vi "Main.vi"() -> ()   [LabVIEW 2017]
panel:
  out "max V":dbl
  out "Loop Iterations":i32
  out "Displacement Array":dbl[](array[numeric])
  out "Velocity Array":dbl[](array[numeric])
  out "Accel Array":dbl[](array[numeric])
  out "Displacement":dbl[](graph)
  out "Velocity":dbl[](graph)
  out "Acceleration":dbl[](graph)
  out "Motion Planning Outputs":T1
  in  "Motion Planning Inputs":T2
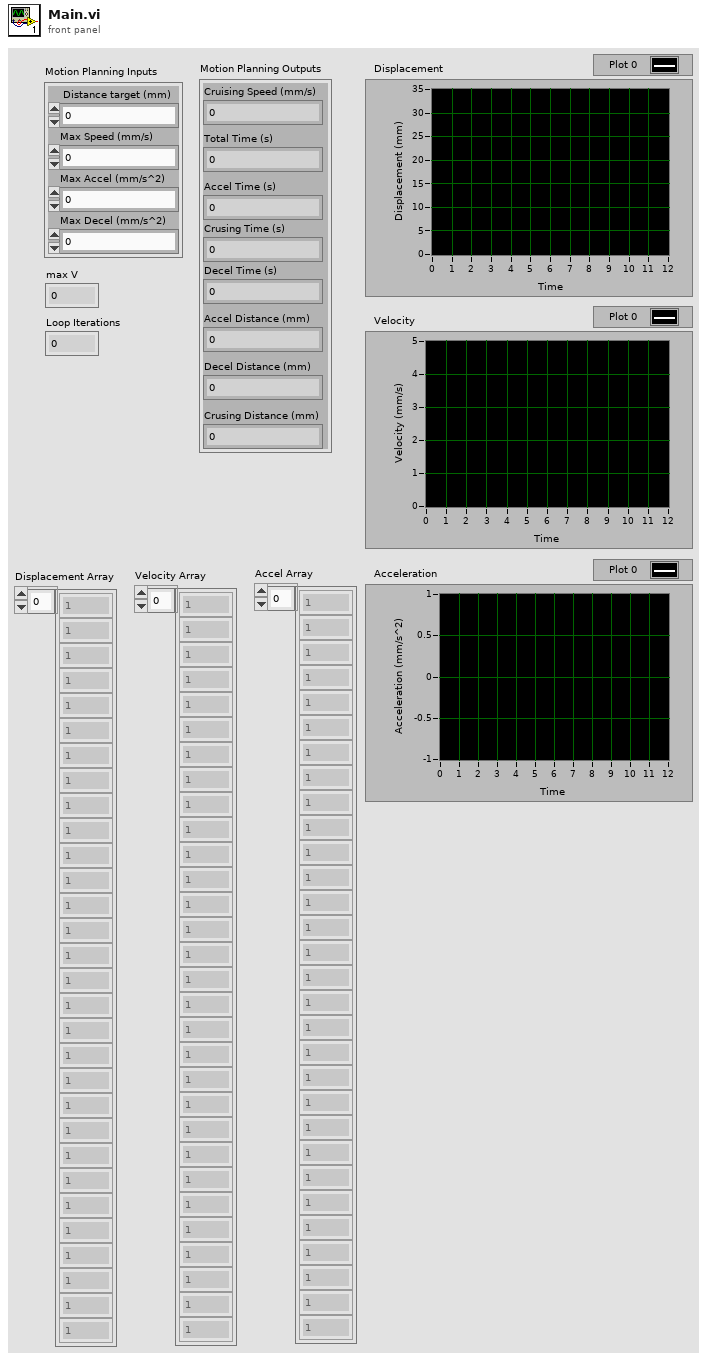
[diagram p1: front panel]
types:
  T1 = cluster{"Cruising Speed (mm/s)":dbl, "Crusing Time (s)":dbl, "Decel Time (s)":dbl, "Accel Time (s)":dbl, "Total Time (s)":dbl, "Accel Distance (mm)":dbl, "Decel Distance (mm)":dbl, "Crusing Distance (mm)":dbl}
  T2 = cluster{" Distance target (mm)":dbl, "Max Accel (mm/s^2)":dbl, "Max Decel (mm/s^2)":dbl, "Max Speed (mm/s) ":dbl}
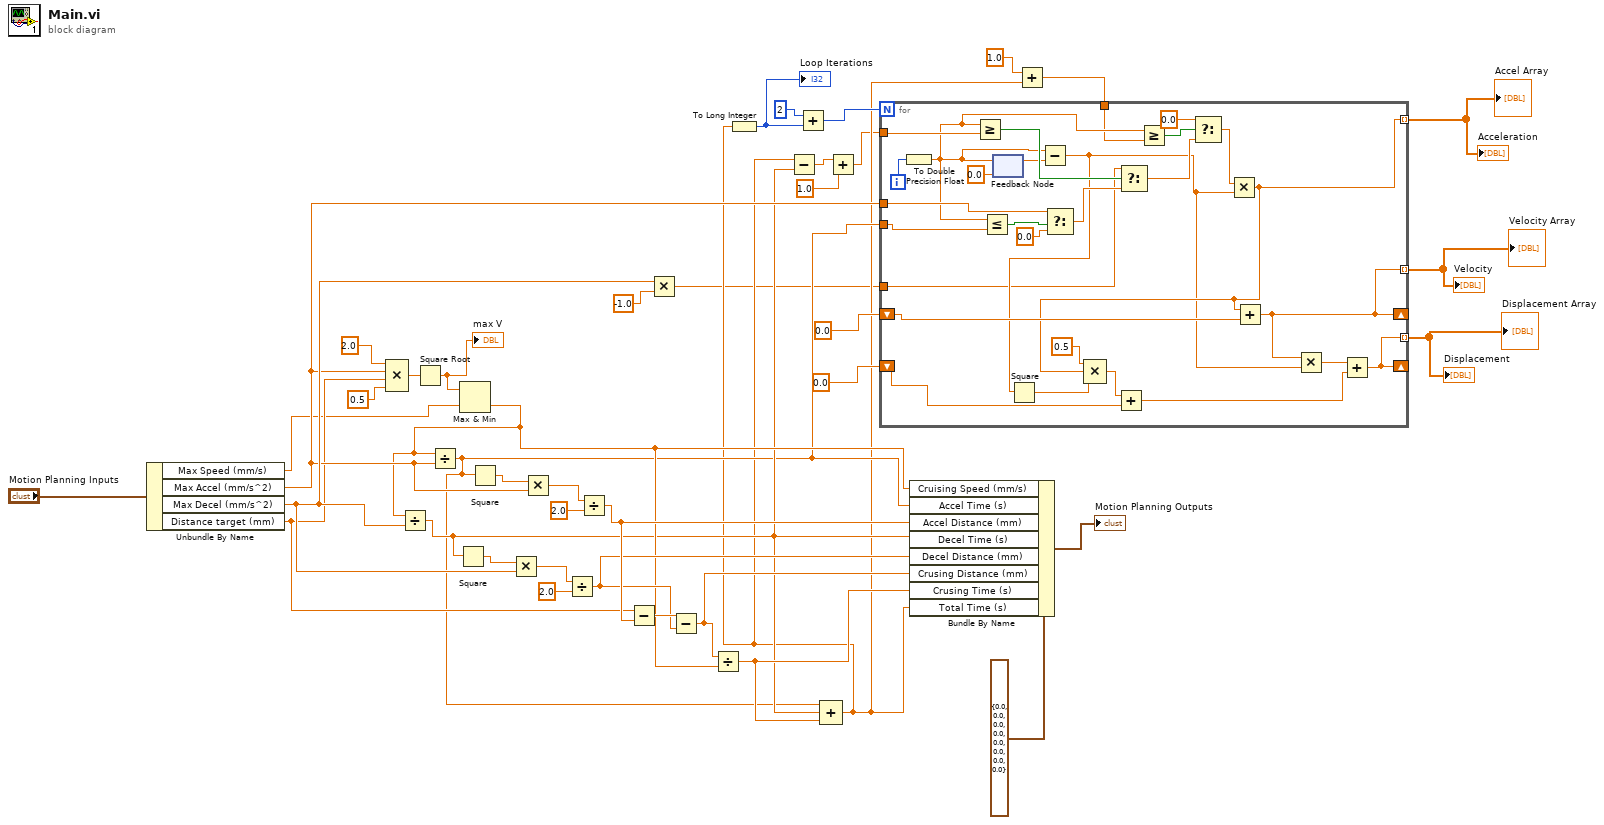
[diagram p0: block diagram]
diagram:
  n1 = Unbundle By Name("Motion Planning Inputs") -> ("Max Speed (mm/s)"=w12:dbl, "Max Accel (mm/s^2)"=w17:dbl, "Max Decel (mm/s^2)"=w26:dbl, "Distance target (mm)"=w16:dbl)
  n2 = Compound Arithmetic op=MULTIPLY(2.0 ("value"), w17, w16, 0.5 ("value")) -> (w14:dbl)
  n3 = Square Root(x=w14) -> (sqrt(x)=w13:dbl)
  "max V" <- w13
  n4 = Max & Min(x=w13, y=w12) -> (min(x,y)=w11:dbl)  [unwired: 1 out]
  n5 = Divide(x=w11, y=w26) -> (x/y=w10:dbl)
  n6 = Divide(x=w11, y=w17) -> (x/y=w9:dbl)
  n7 = Square(x=w10) -> (x^2=w29:dbl)
  n8 = Square(x=w9) -> (x^2=w30:dbl)
  n9 = Multiply(x=w29, y=w26) -> (x*y=w28:dbl)
  n10 = Multiply(x=w30, y=w17) -> (x*y=w31:dbl)
  n11 = Divide(x=w28, y=2.0) -> (x/y=w23:dbl)
  n12 = Divide(x=w31, y=2.0) -> (x/y=w24:dbl)
  n13 = Subtract(x=w16, y=w24) -> (x-y=w25:dbl)
  n14 = Multiply(x=w26, y=-1.0) -> (x*y=w5:dbl)
  n15 = Subtract(x=w25, y=w23) -> (x-y=w22:dbl)
  n16 = Divide(x=w22, y=w11) -> (x/y=w21:dbl)
  n17 = Compound Arithmetic op=ADD(w9, w10, w21) -> (w7:dbl)
  n18 = To Long Integer(number=w7) -> (32bit integer=w34:i32)
  "Loop Iterations" <- w34
  n19 = Subtract(x=w7, y=w10) -> (x-y=w8:dbl)
  n20 = Add(x=2, y=w34) -> (x+y=w20:i32)
  n21 = Add(x=w8, y=1.0) -> (x+y=w2:dbl)
  n22 = Bundle By Name(cluster=T1 {"Cruising Speed (mm/s)"=0.0, "Crusing Time (s)"=0.0, "Decel Time (s)"=0.0, "Accel Time (s)"=0.0, "Total Time (s)"=0.0, "Accel Distance (mm)"=0.0, "Decel Distance (mm)"=0.0, "Crusing Distance (mm)"=0.0} ("Motion Planning Outputs 2"), "Cruising Speed (mm/s)"=w11, "Accel Time (s)"=w9, "Accel Distance (mm)"=w24, "Decel Time (s)"=w10, "Decel Distance (mm)"=w23, "Crusing Distance (mm)"=w22, "Crusing Time (s)"=w21, "Total Time (s)"=w7) -> (→"Motion Planning Outputs":T1)
  n23 = Add(x=1.0, y=w7) -> (x+y=w4:dbl)
  n24 = for {
    N: w20 -> [_]
    tunnel: w17 -> [w67]
    tunnel: [w48] -> w37 mode=indexing
    shift-right: [w45] -> _
    shift-left: 0.0 -> [w64]
    tunnel: [w45] -> w36 mode=indexing
    shift-right: [w60] -> _
    shift-left: 0.0 -> [w59]
    tunnel: [w60] -> w35 mode=indexing
    tunnel: w2 -> [w58]
    tunnel: w9 -> [w57]
    tunnel: w4 -> [w54]
    tunnel: w5 -> [w42]
    i -> [w56]
    n25 = To Double Precision Float(number=w56) -> (double precision float=w55:dbl)
    n26 = Greater Or Equal?(x=w55, y=w58) -> (x >= y?=w66:bool)
    n27 = Less Or Equal?(x=w55, y=w57) -> (x <= y?=w69:bool)
    n28 = feedback-in #1(w55) -> ()
    n29 = feedback #1(0.0) -> (w63:dbl)
    n30 = Subtract(x=w55, y=w63) -> (x-y=w44:dbl)
    n31 = Square(x=w44) -> (x^2=w47:dbl)
    n32 = Select(t=w67, s=w69, f=0.0) -> (s? t:f=w65:dbl)
    n33 = Select(t=w42, s=w66, f=w65) -> (s? t:f=w51:dbl)
    n34 = Greater Or Equal?(x=w55, y=w54) -> (x >= y?=w53:bool)
    n35 = Select(t=0.0, s=w53, f=w51) -> (s? t:f=w50:dbl)
    n36 = Multiply(x=w50, y=w44) -> (x*y=w48:dbl)
    n37 = Compound Arithmetic op=MULTIPLY(0.5 ("value"), w48, w47) -> (w46:dbl)
    n38 = Add(x=w46, y=w59) -> (x+y=w61:dbl)
    n39 = Add(x=w48, y=w64) -> (x+y=w45:dbl)
    n40 = Multiply(x=w45, y=w44) -> (x*y=w43:dbl)
    n41 = Add(x=w43, y=w61) -> (x+y=w60:dbl)
  }
  "Acceleration" <- w37
  "Velocity" <- w36
  "Displacement" <- w35
  "Accel Array" <- w37
  "Velocity Array" <- w36
  "Displacement Array" <- w35
